vi "getNumberOfWheels.vi"(8 "error in (no error)":errorcluster, 11 "vehicle in":refnum<class "vehicleGeneric.lvclass">) -> (0 "error out":errorcluster, 2 "numberOfWheels":dbl, 3 "vehicle out":refnum<class "vehicleGeneric.lvclass">)   [LabVIEW 2011, in "vehicleGeneric.lvclass"]
doc: "This returns the number of wheels in the vehicle."
uses:
  vehicleGeneric.lvclass
  vehicleGeneric.lvclass/vehicleGeneric.ctl
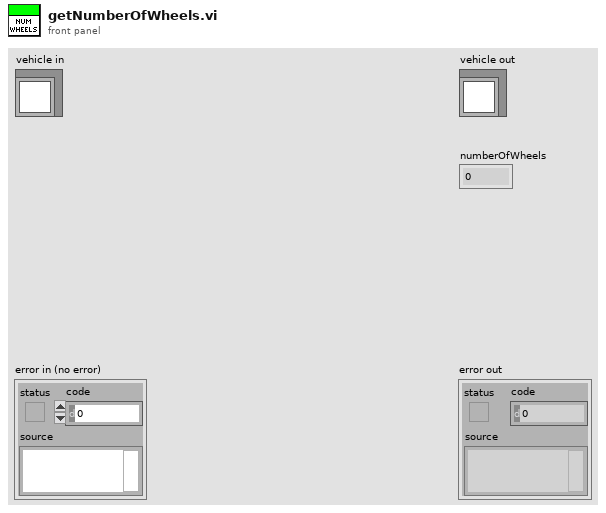
[diagram p1: front panel]
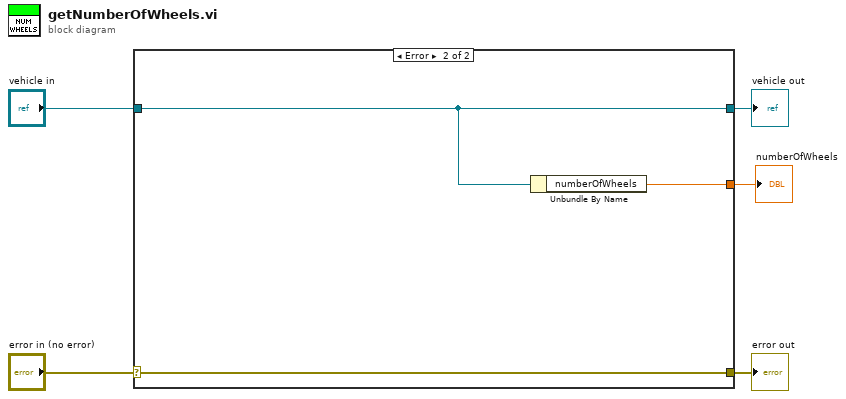
[diagram p0: block diagram]
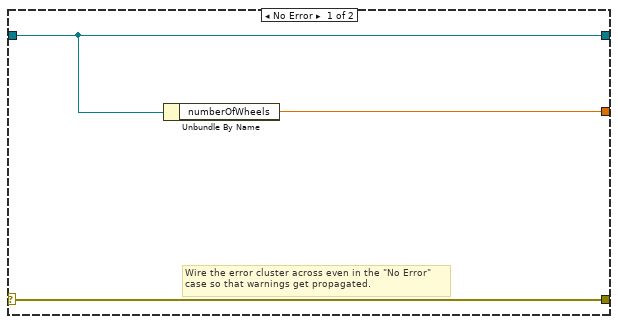
[diagram p2: hidden frame]
diagram:
  n1 = case shown="Error" "error in (no error)" {
    selector: "error in (no error)" -> [w8 w11]
    tunnel: [w8 w11] -> w4
    tunnel: [w7 w10] -> w2
    tunnel: "vehicle in" -> [w7 w10]
    tunnel: [w6 w9] -> w1
    frame No Error {
      # "Wire the error cluster across even in the \"No Error\"\ncase so that warnings get propagated."
      n2 = Unbundle By Name(w7) -> ("numberOfWheels"=w6:dbl)
    }
    frame Error {
      n3 = Unbundle By Name(w10) -> ("numberOfWheels"=w9:dbl)
    }
  }
  "error out" <- w4
  "vehicle out" <- w2
  "numberOfWheels" <- w1
